vi "Timer_INI.vi"(8 "error in (no error)":errorcluster caption="错误输入（无错误）", 11 "Timer 输入":refnum<class "Timer.lvclass">) -> (0 "error out":errorcluster caption="错误输出", 3 "Timer 输出":refnum<class "Timer.lvclass">)   [LabVIEW 2019, in "Timer.lvclass"]
uses:
  Timer.lvclass
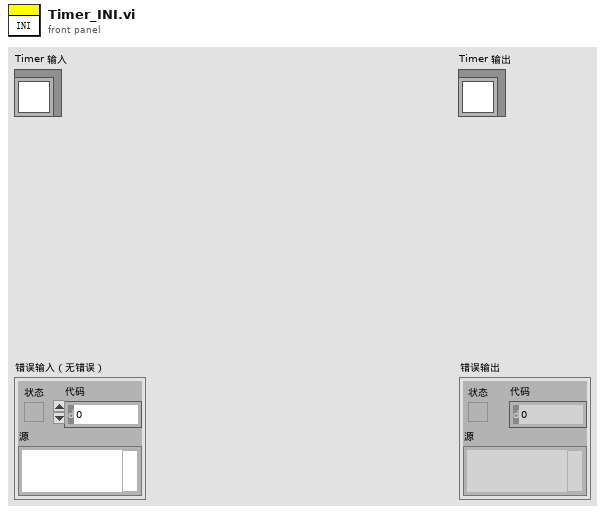
[diagram p1: front panel]
types:
  T1 = typedef "Timer.lvclass/Attribute.ctl" = cluster{"计时？":bool, "计时 (ms)":u32, "停止通知":refnum<notifier>}
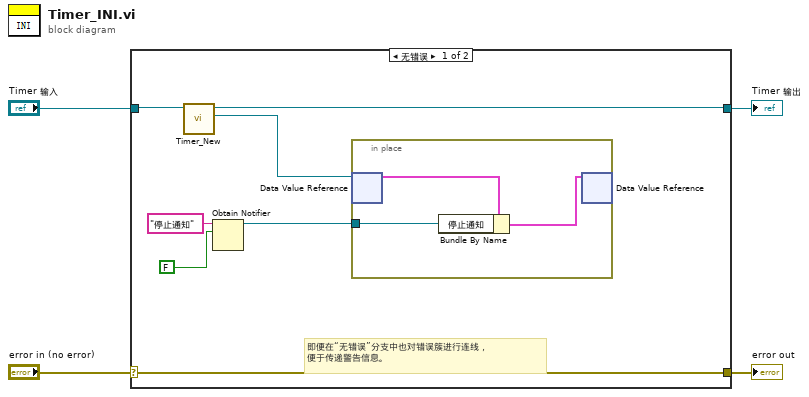
[diagram p0: block diagram]
diagram:
  n1 = case shown="无错误" "error in (no error)" {
    selector: "error in (no error)" -> [w11 w16]
    tunnel: [w11 w16] -> w3
    tunnel: [w9 w15] -> w1
    tunnel: "Timer 输入" -> [w10 w15]
    frame No Error {
      # "即便在“无错误”分支中也对错误簇进行连线，\n便于传递警告信息。"
      n2 = call "Timer_New.vi"("Timer 输入"=w10) -> ("值引用"=w8:refnum<data-value>, "Timer 输出"=w9:refnum<class "Timer.lvclass">)  [unwired: 8 in, 1 out]
      n3 = Obtain Notifier(name (unnamed)="停止通知" ("名称（未命名）"), notification data type=FALSE) -> (notifier out=w6:refnum<notifier>)  [unwired: 2 in, 2 out]
      n4 = in-place {
        in-place-border: w6 -> [w13]
        n5 = in-place-dvr #1(w8) -> (w14:T1)  [unwired: 1 out]
        n6 = Bundle By Name(cluster=w14, "停止通知"=w13) -> (w12:T1)
        n7 = in-place-dvr #1(w12) -> ()  [unwired: 2 out]
      }
    }
    frame Error {
    }
  }
  "error out" <- w3
  "Timer 输出" <- w1
